vi "IEPE - Continuous  Input_tet.vi"() -> ()   [LabVIEW 2025]
doc: "This example demonstrates how to continuously acquire buffered acceleration, sound pressure, or force measurements from IEPE sensors using a DAQmx device.\n\nFor instructions on how to connect your signals to the DAQ device, refer to your device documentation."
uses:
  <vilib>/Math Plots/3D Math Plots/3D Contour/3D Contour XCtrl/3D Contour.xctl
  <vilib>/Utility/error.llb/DialogType.ctl
  <vilib>/DAQmx/read.llb/DAQmx Read (Analog 1D Wfm NChan NSamp).vi
  <extravilib>/ChannelInstances/Tag-bool/Read With Abort.vi
  <extravilib>/ChannelInstances/Tag-bool/Write With Abort.vi
  <vilib>/DAQmx/create/channels.llb/DAQmx Create Channel (AI-Acceleration-Accelerometer).vi
  <vilib>/DAQmx/miscellaneous.llb/DAQmx Fill In Error Info.vi
  <extravilib>/ChannelInstances/Tag-bool/Instantiate.vi
  <extravilib>/ChannelInstances/Tag-bool/EndpointRead.vi
  <vilib>/Waveform/WDTOps.llb/WDT Append Waveforms DBL.vi
  <extravilib>/ChannelInstances/Tag-bool/Endpoint.vi
  <vilib>/DAQmx/configure/timing.llb/DAQmx Timing (Sample Clock).vi
  <vilib>/DAQmx/configure/task.llb/DAQmx Configure Logging (TDMS).vi
  <vilib>/DAQmx/create/channels.llb/DAQmx Create Channel (AI-Sound Pressure-Microphone).vi
  <vilib>/DAQmx/create/channels.llb/DAQmx Create Channel (AI-Force-IEPE Sensor).vi
  <vilib>/DAQmx/configure/trigger.llb/DAQmx Start Trigger (Analog Edge).vi
  <vilib>/DAQmx/configure/trigger.llb/DAQmx Start Trigger (Time).vi
  <vilib>/DAQmx/configure/trigger.llb/DAQmx Start Trigger (Digital Edge).vi
  <vilib>/Waveform/WDTOps.llb/WDT Waveform Duration DBL.vi
  <resource>/objmgr/daqmx.rc
  <extravilib>/ChannelInstances/Tag-bool.lvlib
panel:
  out "_Vib3_3D-Kontur 3":refnum<class "3D Plot Datatype.lvclass">[](xcontrol)
  out "_Vib2_3D-Kontur":refnum<class "3D Plot Datatype.lvclass">[](xcontrol)
  in  "last order plot":sgl
  in  "rotation speed":sgl
  out "_Vib1_3D-Kontur":refnum<class "3D Plot Datatype.lvclass">[](xcontrol)
  in  "filename":string
  in  "Root folder":path
  in  "on hold time (s)":u32=900
  out "FFT":cluster{dbl, "freq_step":dbl, "abs_FFT":dbl[]}[](graph)
  in  "duration (s) control":dbl=30.0
  out "current duration":dbl caption="Dauer" format="%0.2f"
  in  "Trigger Type":T1(tab)
  in  "Digital Start Trigger Edge":i32(ring)=10280 caption="Edge" items=["Rising"=10280, "Falling"=10171]
  in  "Digital Start Trigger Source":tag="/Dev1/PFI0" caption="Source"
  in  "Digital Pause Trigger Pause When":i32(ring)=10192 caption="Pause When" items=["High"=10192, "Low"=10214]
  in  "Digital Pause Trigger Source":tag="/Dev1/PFI0" caption="Source"
  in  "Analog Start Trigger Level":dbl caption="Level" format="%0.2f"
  in  "Analog Start Trigger Hysteresis":dbl caption="Hysteresis" format="%.2f"
  in  "Analog Start Trigger Slope":i32(ring)=10280 caption="Slope" items=["Rising"=10280, "Falling"=10171]
  in  "Analog Start Trigger Source":string="APFI0" caption="Source"
  in  "Analog Pause Trigger Source":string="APFI0" caption="Source"
  in  "Analog Pause Trigger Pause When":i32(ring)=10093 caption="Pause When" items=["Above Level"=10093, "Below Level"=10107]
  in  "Analog Pause Trigger Level":dbl caption="Level" format="%.2f"
  in  "When":timestamp
  in  "Select Time\nManually":bool
  in  "IEPE Current Value (A)":dbl=0.004
  in  "IEPE Excitation Source":i32(ring)=10200 items=["Internal"=10200, "External"=10167, "None"=10230]
  in  "Terminal Configuration":i32(ring)=-1 items=["default"=-1, "RSE"=10083, "NRSE"=10078, "Differential"=10106, "Pseudodifferential"=12529]
  in  "Physical Channel":tag="cDAQ3Mod2/ai0"
  in  "Task Type":T2(tab)
  in  "Min Acceleration":dbl=-100.0
  in  "Max Acceleration":dbl=100.0
  in  "Sensitivity":dbl=50.0
  in  "Acceleration Units":i32(ring)=10186 items=["g"=10186, "m/s^2"=12470, "in/s^2"=12471, "From Custom Scale"=10065]
  in  "Sensitivity Units":i32(ring)=12509 items=["mVolts/g"=12509, "Volts/g"=12510]
  in  "Max Sound Pressure Level (dB)":dbl=120.0
  in  "Sound Pressure Units":i32(ring)=10081 items=["Pascals"=10081, "From Custom Scale"=10065]
  in  "Microphone Sensitivity":dbl=10.0
  in  "Sensitivity":dbl=50.0
  in  "Min Force":dbl=-100.0
  in  "Max Force":dbl=100.0
  in  "Sensitivity Units":i32(ring)=15891 items=["mVolts/N"=15891, "mVolts/lb"=15892]
  in  "Force Units":i32(ring)=15875 items=["Newtons"=15875, "Pounds"=15876, "From Custom Scale"=10065]
  in  "Stop":bool
  out "Waveform Graph":waveform(dbl)[](graph)
  in  "TDMS File Path":path
  in  "Samples per Loop":i32=100
  in  "Sample Rate":dbl=1000.0
  in  "Sample Clock Source":tag="OnboardClock"
  out "Actual Sample Rate":dbl=1000.0000111176631 format="%0.2f"
  in  "Logging Mode":i32(ring)=10231 items=["Off"=10231, "Log and Read"=15842]
  # "Channel Settings"
  # "Acquired Data"
  # "Trigger Settings"
  # "Timing Settings"
  # "Logging Settings"
  # "To enable triggers, select a tab above, and configure the settings.\n\nNot all hardware supports all trigger types. Refer to your device documentation for more information."
  # "This trigger type is not supported in continuous sample timing. \n\nRefer to your device documentation for more information on which triggers are supported."
  # "This trigger type is not supported in continuous sample timing. \n\nRefer to your device documentation for more information on which triggers are supported."
  # "If time is not manually set, task will begin after 10 seconds"
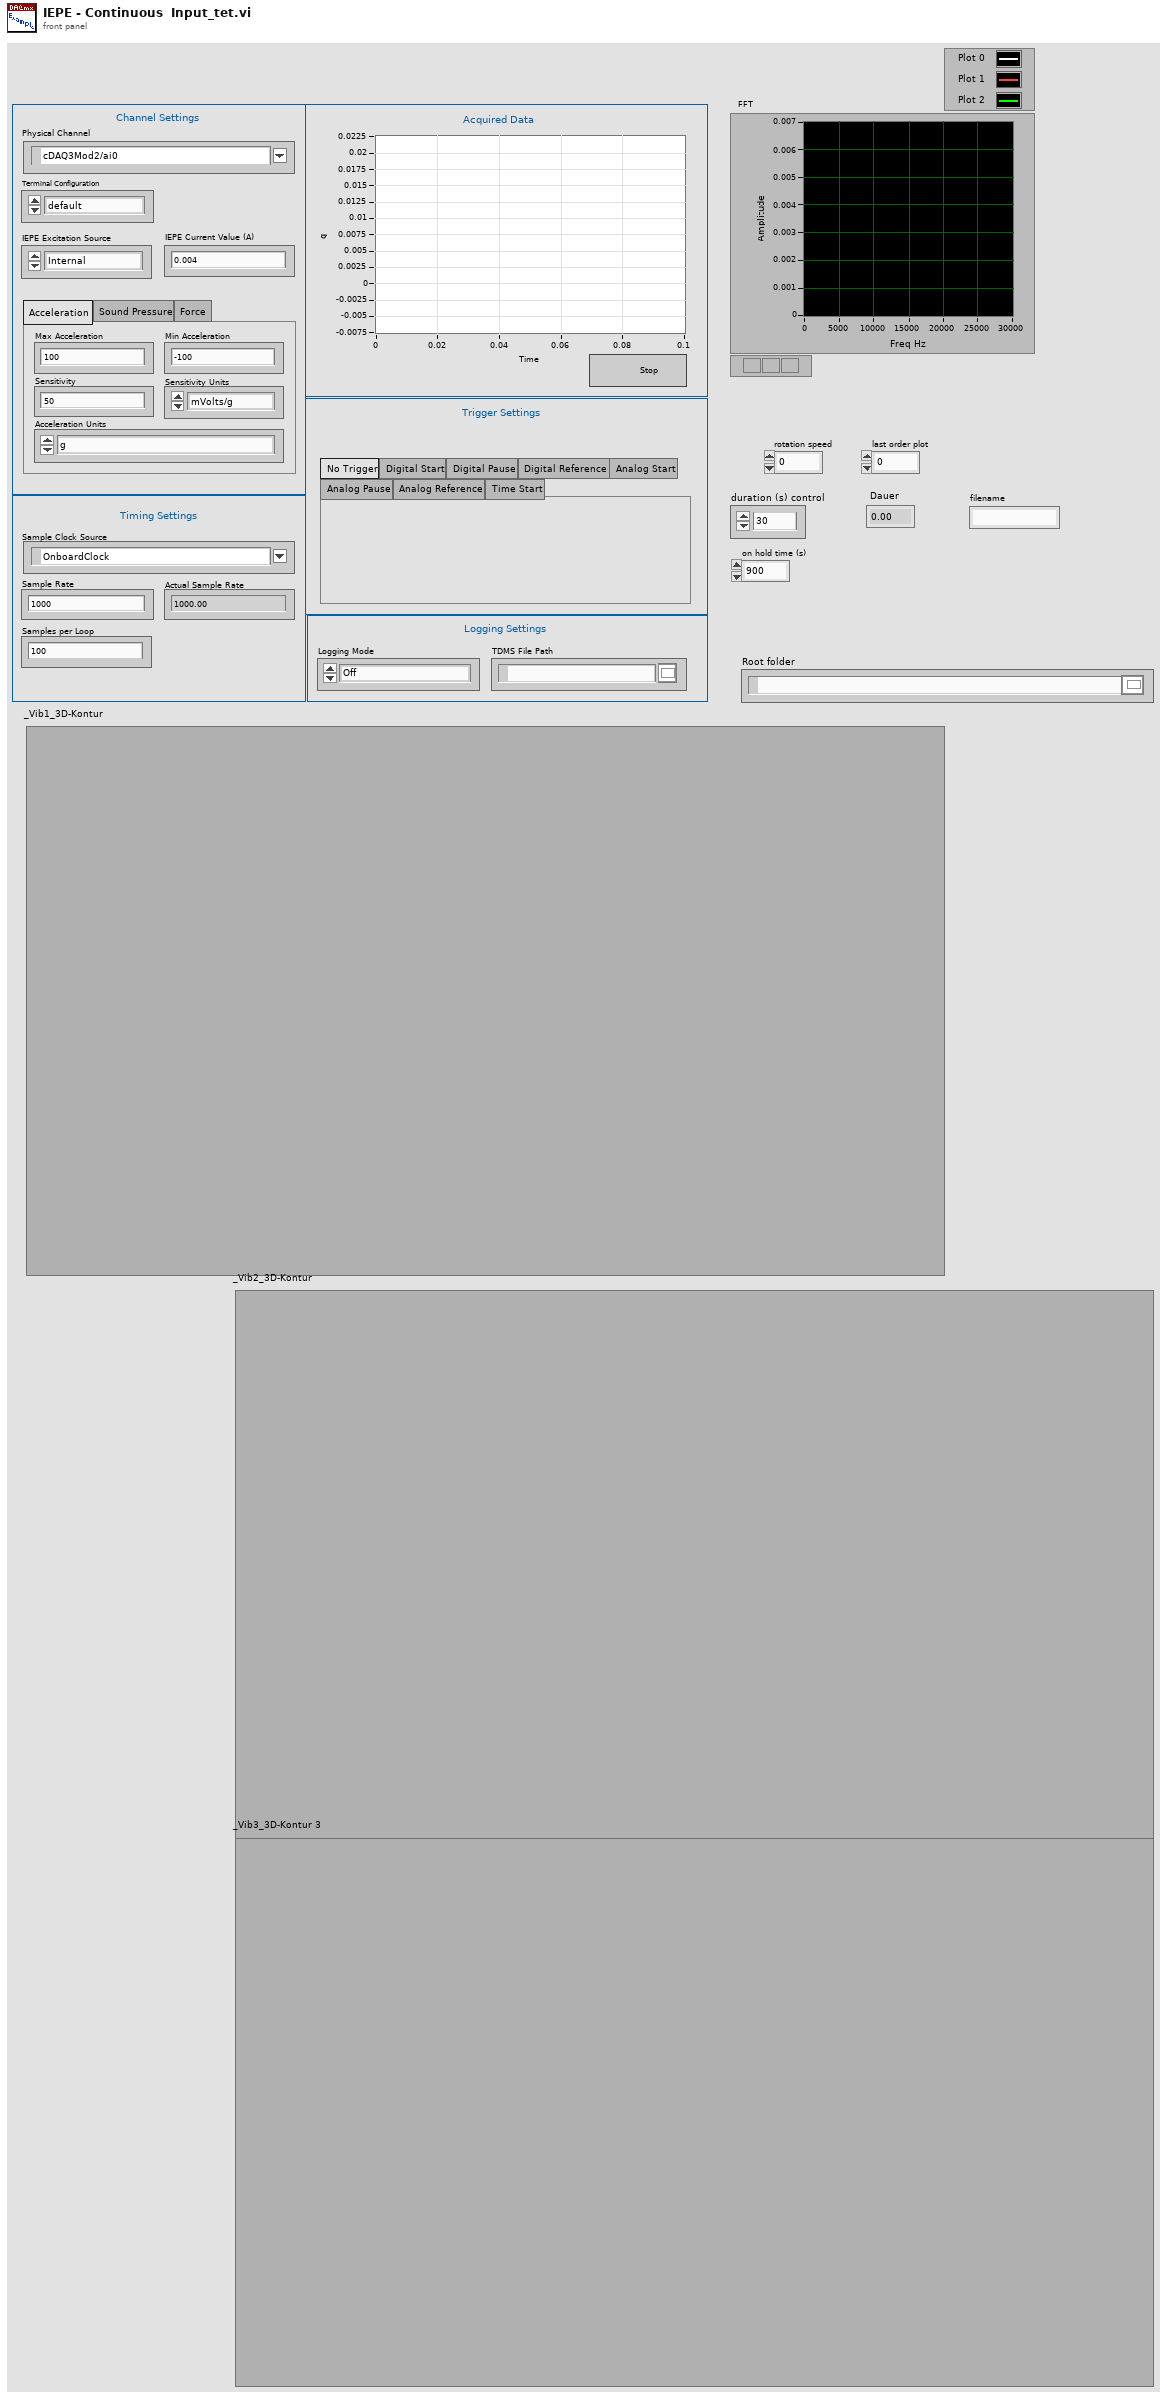
[diagram p1: front panel]
types:
  T1 = enum32{"No Trigger", "Digital Start", "Digital Pause", "Digital Reference", "Analog Start", "Analog Pause", "Analog Reference", "Time Start"}
  T2 = enum32{"Acceleration", "Sound Pressure", "Force"}
  T3 = cluster{"abs_FFT":dbl[], "frequencies":dbl[], "Huell_spec":dbl[], "Envelope":dbl[], "freq_step":dbl, "duration":dbl}
  T4 = typedef "DialogType.ctl" = u16
  T5 = cluster{"abs_FFT":dbl[], "frequencies":dbl[], "Huell_spec":dbl[], "Envelope":dbl[], "freq_step":dbl, "duration":dbl}[]
  T6 = typedef "Tag-bool.lvlib/))Channel.ctl" = refnum<queue>
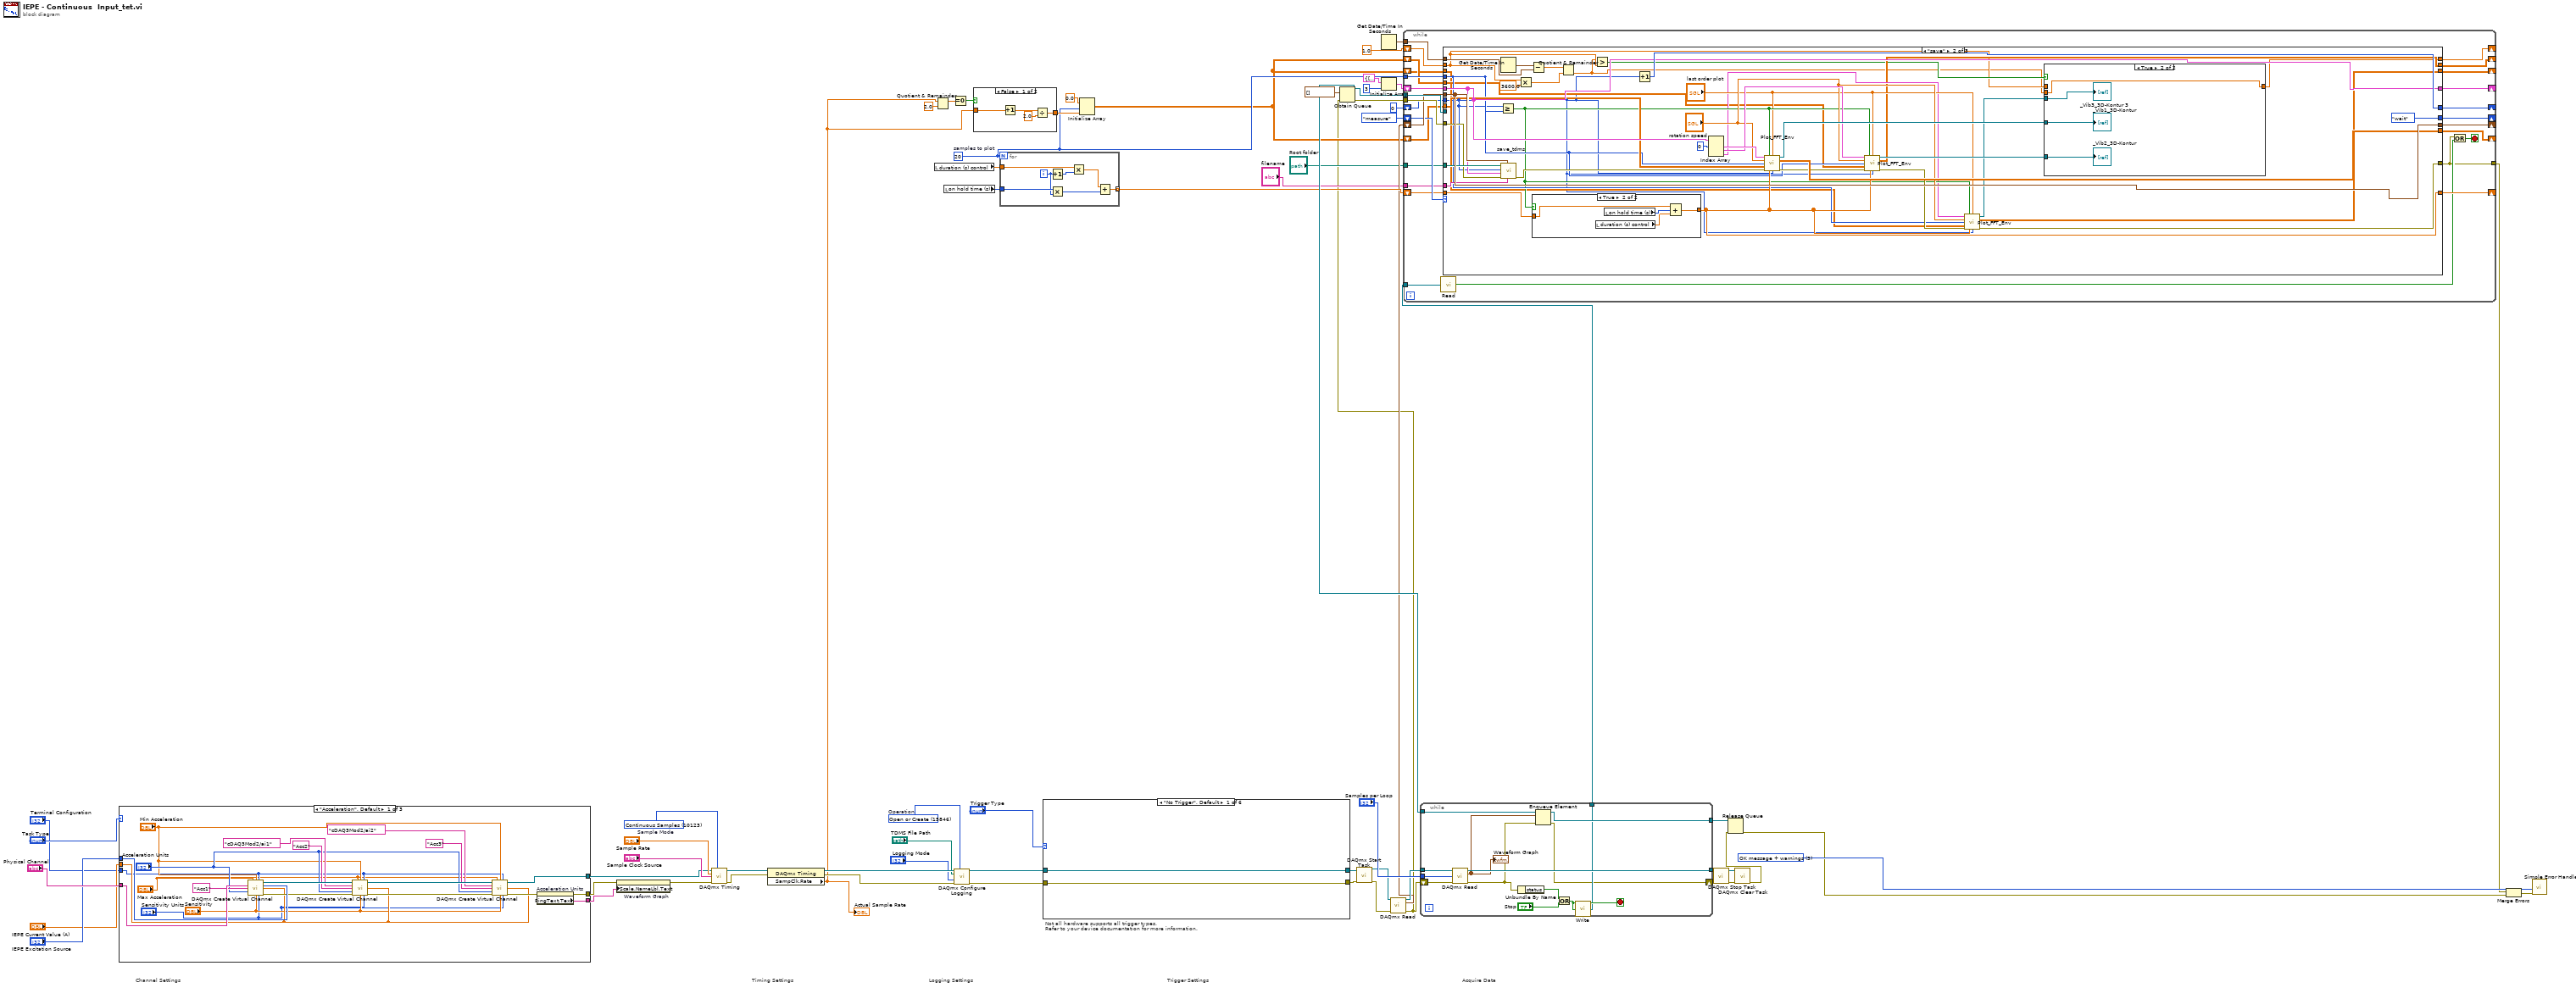
[diagram p0: block diagram]
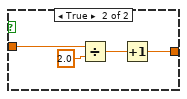
[diagram p2: hidden frame]
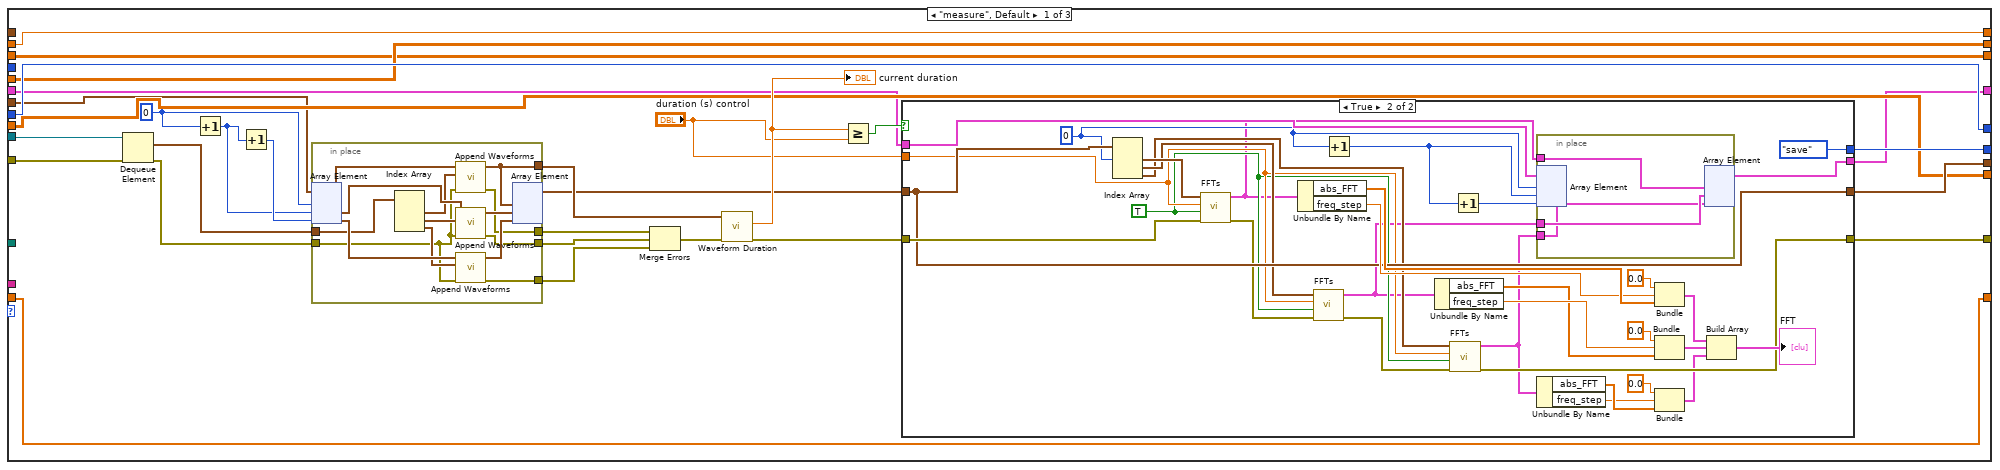
[diagram p3: hidden frame]
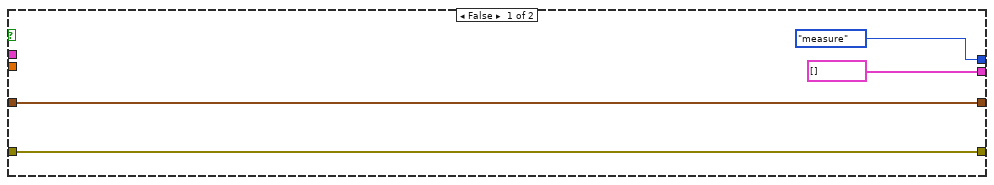
[diagram p4: hidden frame]
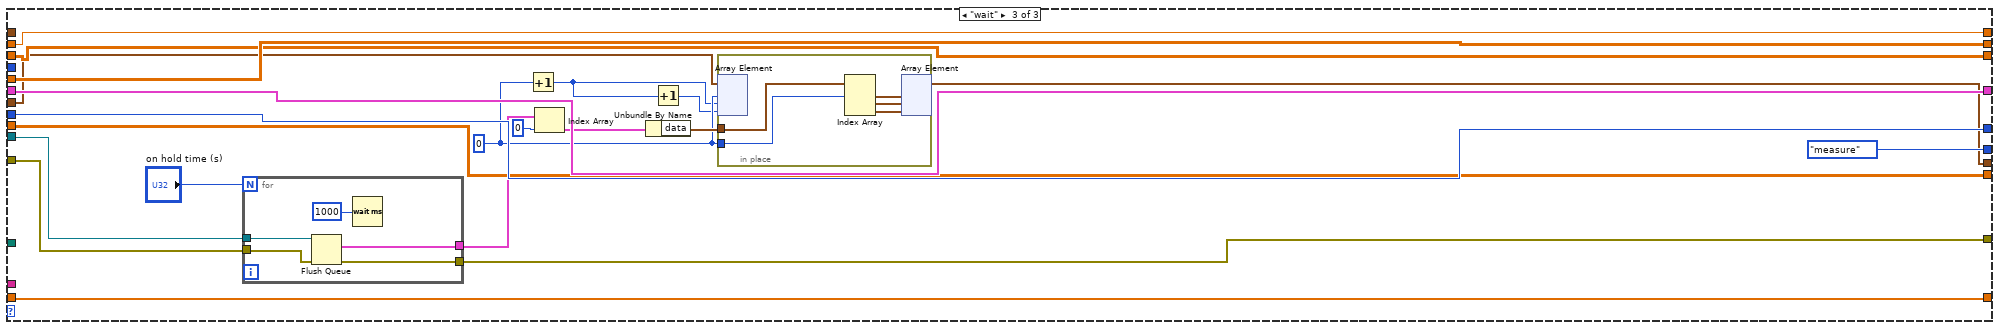
[diagram p7: hidden frame]
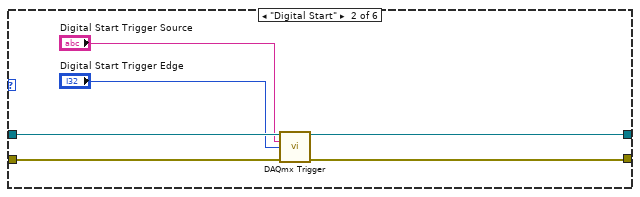
[diagram p8: hidden frame]
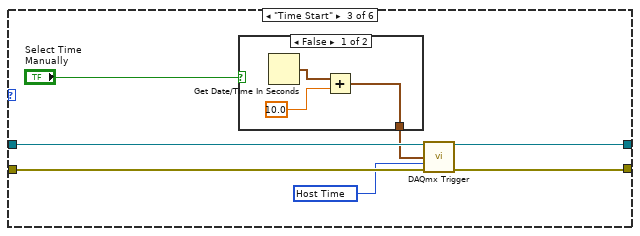
[diagram p9: hidden frame]
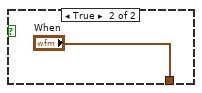
[diagram p10: hidden frame]
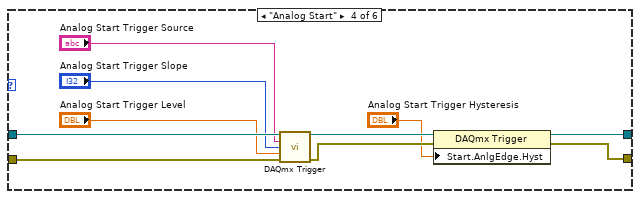
[diagram p11: hidden frame]
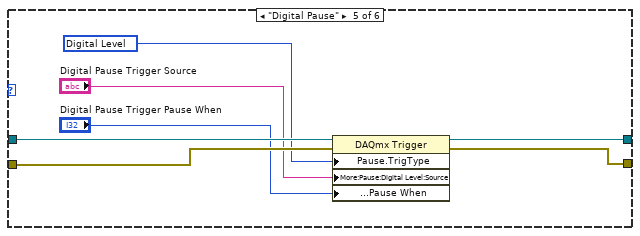
[diagram p12: hidden frame]
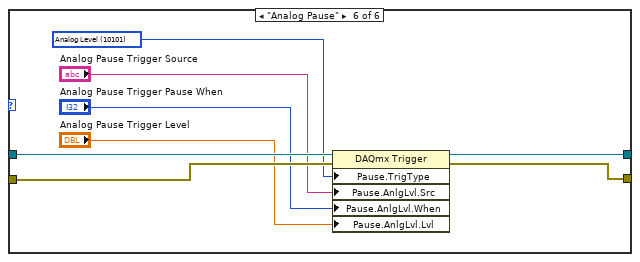
[diagram p13: hidden frame]
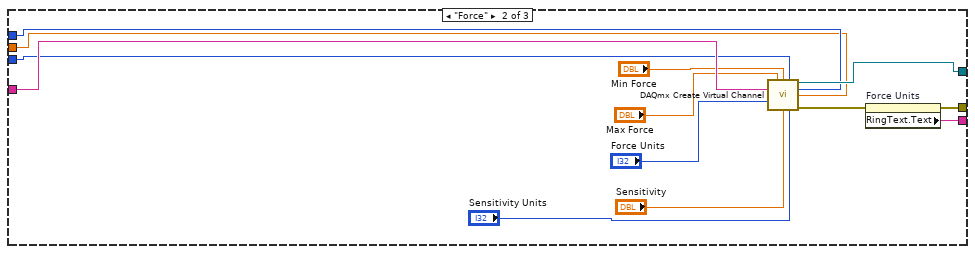
[diagram p14: hidden frame]
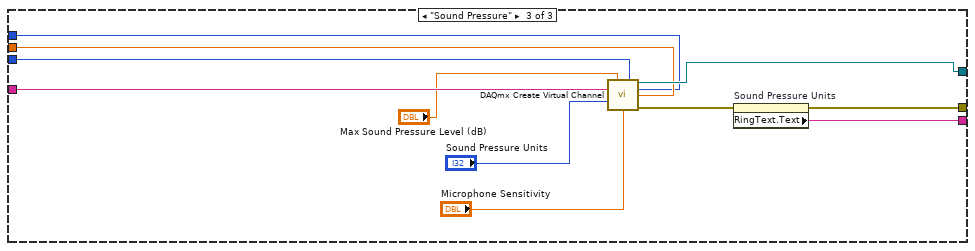
[diagram p15: hidden frame]
diagram:
  w14 = 20  # samples to plot
  w41 = T4 3 items=["no dialog", "OK message", "continue or stop message", "OK message + warnings", "continue/stop + warnings"] ("type of dialog (OK msg:1)")
  w59 = 15846 items=["Open"=10437, "Open or Create"=15846, "Create or Replace"=15847, "Create"=15848]  # Operation
  w62 = 10123 items=["Finite Samples"=10178, "Continuous Samples"=10123, "Hardware Timed Single Point"=12522]  # Sample Mode
  # "Trigger Settings"
  # "Not all hardware supports all trigger types.\nRefer to your device documentation for more information."
  # "Acquire Data"
  # "Timing Settings"
  # "Channel Settings"
  # "Logging Settings"
  n1 = case shown="\"Acceleration\", Default" "Task Type" {
    tunnel: [w84 w89 w103] -> w48
    tunnel: [w77 w99 w110] -> w49
    tunnel: "Physical Channel" -> [w86 w98 w109]
    tunnel: "IEPE Excitation Source" -> [w85 w97 w105]
    tunnel: "IEPE Current Value (A)" -> [w73 w96 w106]
    tunnel: "Terminal Configuration" -> [w66 w95 w108]
    tunnel: [w83 w88 w102] -> w47
    frame "Acceleration", Default {
      n2 = call-poly <vilib>:"DAQmx Create Virtual Channel.vi"("maximum value"="Max Acceleration", "minimum value"="Min Acceleration", "input terminal configuration"=w66, "physical channels"=w86, "current excitation source"=w85, "name to assign"="Acc1", "current excitation value"=w73, "units"="Acceleration Units", "sensitivity"="Sensitivity", "sensitivity units"="Sensitivity Units") -> ("task out"=w81:refnum<k21>, "error out"=w80:errorcluster)  [unwired: 4 in]
      n3 = call-poly <vilib>:"DAQmx Create Virtual Channel.vi"("task in"=w81, "maximum value"="Max Acceleration", "minimum value"="Min Acceleration", "input terminal configuration"=w66, "physical channels"=tag "cDAQ3Mod2/ai1" ("Physical Channel 2"), "name to assign"="Acc2", "current excitation value"=w73, "units"="Acceleration Units", "error in"=w80, "sensitivity"="Sensitivity", "sensitivity units"="Sensitivity Units") -> ("task out"=w79:refnum<k21>, "error out"=w78:errorcluster)  [unwired: 3 in]
      n4 = call-poly <vilib>:"DAQmx Create Virtual Channel.vi"("task in"=w79, "maximum value"="Max Acceleration", "minimum value"="Min Acceleration", "input terminal configuration"=w66, "physical channels"=tag "cDAQ3Mod2/ai2" ("Physical Channel 2"), "name to assign"="Acc3", "current excitation value"=w73, "units"="Acceleration Units", "error in"=w78, "sensitivity"="Sensitivity", "sensitivity units"="Sensitivity Units") -> ("task out"=w77:refnum<k21>, "error out"=w76:errorcluster)  [unwired: 3 in]
      n5 = property on="Acceleration Units" class="Ring (strict)"(error in=w76) -> (error out=w84:errorcluster, "RingText.Text"=w83:string)  [unwired: 1 in, 1 out]
    }
    frame "Force" {
      n6 = call-poly <vilib>:"DAQmx Create Virtual Channel.vi"("maximum value"="Max Force", "minimum value"="Min Force", "input terminal configuration"=w95, "physical channels"=w98, "current excitation source"=w97, "current excitation value"=w96, "units"="Force Units", "sensitivity"="Sensitivity", "sensitivity units"="Sensitivity Units") -> ("task out"=w99:refnum<k21>, "error out"=w87:errorcluster)  [unwired: 5 in]
      n7 = property on="Force Units" class="Ring (strict)"(error in=w87) -> (error out=w89:errorcluster, "RingText.Text"=w88:string)  [unwired: 1 in, 1 out]
    }
    frame "Sound Pressure" {
      n8 = call-poly <vilib>:"DAQmx Create Virtual Channel.vi"("maximum sound pressure level"="Max Sound Pressure Level (dB)", "input terminal configuration"=w108, "physical channels"=w109, "current excitation source"=w105, "current excitation value"=w106, "units"="Sound Pressure Units", "microphone sensitivity"="Microphone Sensitivity") -> ("task out"=w110:refnum<k21>, "error out"=w101:errorcluster)  [unwired: 7 in]
      n9 = property on="Sound Pressure Units" class="Ring (strict)"(error in=w101) -> (error out=w103:errorcluster, "RingText.Text"=w102:string)  [unwired: 1 in, 1 out]
    }
  }
  n10 = property on="Waveform Graph" class="WFGraph (strict)"(error in=w48, "YScale.NameLbl.Text"=w47) -> (error out=w46:errorcluster)  [unwired: 1 in, 1 out]
  n11 = call-poly <vilib>:"DAQmx Timing.vi"("task/channels in"=w49, "sample mode"=w62, "rate"="Sample Rate", "source"="Sample Clock Source", "error in"=w46) -> ("task out"=w64:refnum<k21>, "error out"=w63:errorcluster)  [unwired: 9 in]
  n12 = property class="DAQmx Timing"(reference=w64, error in=w63) -> (reference out=w61:refnum<k21>, error out=w60:errorcluster, "SampClk.Rate"=w24:dbl)
  "Actual Sample Rate" <- w24
  n13 = local read "duration (s) control"() -> (w16:dbl)
  n14 = Quotient & Remainder(x=w24, y=2.0) -> (x-y*floor(x/y)=w25:dbl)  [unwired: 1 out]
  n15 = local read "on hold time (s)"() -> (w17:u32)
  n16 = Equal To 0?(x=w25) -> (x = 0?=w26:bool)
  n17 = call-poly <vilib>:"DAQmx Configure Logging.vi"("task/channels in"=w61, "operation"=w59, "file path"="TDMS File Path", "logging mode"="Logging Mode", "error in"=w60) -> ("task out"=w38:refnum<k21>, "error out"=w39:errorcluster)  [unwired: 9 in]
  n18 = case shown="False" w26 {
    tunnel: w24 -> [w113 w116]
    tunnel: [w111 w115] -> w23
    frame False {
      n19 = Increment(x=w113) -> (x+1=w112:dbl)
      n20 = Divide(x=w112, y=2.0) -> (x/y=w111:dbl)
    }
    frame True {
      n21 = Divide(x=w116, y=2.0) -> (x/y=w118:dbl)
      n22 = Increment(x=w118) -> (x+1=w115:dbl)
    }
  }
  n23 = for {
    N: w14 -> [_]
    tunnel: w17 -> [w125]
    tunnel: w16 -> [w122]
    tunnel: [w119] -> w15 mode=indexing
    i -> [w124]
    n24 = Increment(x=w124) -> (x+1=w123:i32)
    n25 = Multiply(x=w125, y=w124) -> (x*y=w120:u32)
    n26 = Multiply(x=w122, y=w123) -> (x*y=w121:dbl)
    n27 = Add(x=w121, y=w120) -> (x+y=w119:dbl)
  }
  n28 = case shown="\"No Trigger\", Default" "Trigger Type" {
    tunnel: w38 -> [w127 w133 w140 w154 w161 w169]
    tunnel: w39 -> [w126 w132 w139 w153 w158 w166]
    tunnel: [w127 w131 w138 w151 w160 w168] -> w36
    tunnel: [w126 w130 w137 w150 w159 w167] -> w37
    frame "No Trigger", Default {
    }
    frame "Digital Start" {
      n29 = call-poly <vilib>:"DAQmx Trigger.vi"("task/channels in"=w133, "source"="Digital Start Trigger Source", "edge"="Digital Start Trigger Edge", "error in"=w132) -> ("task out"=w131:refnum<k21>, "error out"=w130:errorcluster)  [unwired: 10 in]
    }
    frame "Time Start" {
      w134 = 16126 items=["Host Time"=16126, "I/O Device Time"=16127] ("timescale")
      n30 = case shown="False" "Select Time\nManually" {
        tunnel: [w142 "When"] -> w135
        frame False {
          n31 = Get Date/Time In Seconds() -> (seconds since 1Jan1904=w143:timestamp)
          n32 = Add(x=w143, y=10.0) -> (x+y=w142:timestamp)
        }
        frame True {
        }
      }
      n33 = call-poly <vilib>:"DAQmx Trigger.vi"("task/channels in"=w140, "when"=w135, "timescale"=w134, "error in"=w139) -> ("task out"=w138:refnum<k21>, "error out"=w137:errorcluster)  [unwired: 10 in]
    }
    frame "Analog Start" {
      n34 = call-poly <vilib>:"DAQmx Trigger.vi"("task/channels in"=w154, "source"="Analog Start Trigger Source", "slope"="Analog Start Trigger Slope", "level"="Analog Start Trigger Level", "error in"=w153) -> ("task out"=w149:refnum<k21>, "error out"=w148:errorcluster)  [unwired: 9 in]
      n35 = property class="DAQmx Trigger"(reference=w149, error in=w148, "Start.AnlgEdge.Hyst"="Analog Start Trigger Hysteresis") -> (reference out=w151:refnum<k21>, error out=w150:errorcluster)
    }
    frame "Digital Pause" {
      w157 = 10152 items=["Analog Level"=10101, "Analog Window"=10103, "Digital Level"=10152, "Digital Pattern"=10398, "None"=10230] ("Pause.TrigType")
      n36 = property class="DAQmx Trigger"(reference=w161, error in=w158, "Pause.TrigType"=w157, "More:Pause:Digital Level:Source"="Digital Pause Trigger Source", "More:Pause:Digital Level:Pause When"="Digital Pause Trigger Pause When") -> (reference out=w160:refnum<k21>, error out=w159:errorcluster)
    }
    frame "Analog Pause" {
      w165 = 10101 items=["Analog Level"=10101, "Analog Window"=10103, "Digital Level"=10152, "Digital Pattern"=10398, "None"=10230] ("Pause.TrigType")
      n37 = property class="DAQmx Trigger"(reference=w169, error in=w166, "Pause.TrigType"=w165, "Pause.AnlgLvl.Src"="Analog Pause Trigger Source", "Pause.AnlgLvl.When"="Analog Pause Trigger Pause When", "Pause.AnlgLvl.Lvl"="Analog Pause Trigger Level") -> (reference out=w168:refnum<k21>, error out=w167:errorcluster)
    }
  }
  n38 = Initialize Array(0.0 ("Element"), w14, w23) -> (w5:dbl[][])
  n39 = call <vilib>:"DAQmx Start Task.vi"("task/channels in"=w36, "error in"=w37) -> ("task out"=w31:refnum<k21>, "error out"=w30:errorcluster)  [unwired: 12 in]
  n40 = Get Date/Time In Seconds() -> (seconds since 1Jan1904=w2:timestamp)
  n41 = Initialize Array(T3 {"abs_FFT"=[], "frequencies"=[], "Huell_spec"=[], "Envelope"=[], "freq_step"=0.0, "duration"=0.0} ("output cluster"), 3 ("dimension size")) -> (w11:T5)
  n42 = call-poly <vilib>:"DAQmx Read.vi"("task/channels in"=w31, "error in"=w30) -> ("task out"=w29:refnum<k21>, "data"=w12:waveform(dbl)[], "error out"=w4:errorcluster)  [unwired: 11 in]
  n43 = Obtain Queue(element data type=waveform(dbl)[] [] ("data"), error in (no error)=w4) -> (queue out=w35:refnum<queue>, error out=w3:errorcluster)  [unwired: 3 in, 1 out]
  n44 = while {
    tunnel: w29 -> [w182]
    tunnel: [w179] -> w43
    tunnel: w35 -> [w175]
    tunnel: [w174] -> w34
    tunnel: "Samples per Loop" -> [w173]
    tunnel: [w172] -> w6
    shift-right: [w170] -> w42
    shift-left: w4 -> [w181]
    stop <- w180 stop-if-true
    n45 = call-poly <vilib>:"DAQmx Read.vi"("task/channels in"=w182, "number of samples per channel"=w173, "error in"=w181) -> ("task out"=w179:refnum<k21>, "data"=w176:waveform(dbl)[], "error out"=w171:errorcluster)  [unwired: 10 in]
    "Waveform Graph" <- w176
    n46 = Unbundle By Name(w171) -> ("status"=w178:bool)
    n47 = Enqueue Element(queue=w175, element=w176, error in (no error)=w171) -> (queue out=w174:refnum<queue>, error out=w170:errorcluster)  [unwired: 1 in, 1 out]
    n48 = Or(x=w178, y="Stop") -> (x .or. y?=w180:bool)
    n49 = call <extravilib>:"Write.vi"("element"=w180) -> ("channel"=w172:T6)  [unwired: 1 out]
  }
  n50 = while {
    tunnel: w35 -> [w210]
    tunnel: w3 -> [w209]
    shift-right: [w208] -> _
    shift-left: w12 -> [w207]
    shift-right: [w194] -> _
    shift-left: w11 -> [w202]
    shift-right: [w205] -> _
    shift-left: enum16{"measure", "save", "wait"}."measure" -> [w206]
    shift-right: [w203] -> _
    shift-left: 0 -> [w204]
    tunnel: [w191] -> w21
    tunnel: "Root folder" -> [w201]
    tunnel: "filename" -> [w200]
    shift-right: [w198] -> _
    shift-left: w5 -> [w199]
    tunnel: w14 -> [w196]
    shift-right: [w195] -> _
    shift-left: w15 -> [w197]
    tunnel: w6 -> [w193]
    shift-right: [w187] -> _
    shift-left: w5 -> [w189]
    shift-right: [w186] -> _
    shift-left: w5 -> [w188]
    tunnel: w2 -> [w185]
    shift-right: [w184] -> _
    shift-left: 1.0 -> [w183]
    stop <- w190 stop-if-true
    n51 = call <extravilib>:"Read.vi"("channel"=w193) -> ("element"=w192:bool)  [unwired: 1 in, 1 out]
    n52 = case shown="\"save\"" w206 {
      tunnel: w210 -> [w239 _ w361]
      tunnel: w209 -> [w238 w327 w362]
      tunnel: [w235 w330 w345] -> w208
      tunnel: [w234 w314 w357] -> w191
      tunnel: w207 -> [w227 w330 w350]
      tunnel: [w214 w322 w358] -> w194
      tunnel: [w232 enum16{"measure", "save", "wait"}."wait" enum16{"measure", "save", "wait"}."measure"] -> w205
      tunnel: w204 -> [w231 w302 w363]
      tunnel: [w231 w331 w363] -> w203
      tunnel: w202 -> [w215 w322 w358]
      tunnel: w201 -> [_ w328 _]
      tunnel: w200 -> [_ w329 _]
      tunnel: w199 -> [w230 w320 w355]
      tunnel: [w230 w319 w355] -> w198
      tunnel: w197 -> [w228 w324 w354]
      tunnel: w196 -> [_ w311 _]
      tunnel: [w228 w312 w354] -> w195
      tunnel: w189 -> [w213 w306 w353]
      tunnel: w188 -> [w212 w305 w352]
      tunnel: [w213 w304 w353] -> w187
      tunnel: [w212 w303 w352] -> w186
      tunnel: w185 -> [_ w300 _]
      tunnel: [w211 w295 w343] -> w184
      tunnel: w183 -> [w211 w294 w343]
      frame "measure", Default {
        w217 = 0
        n53 = Dequeue Element(queue=w239, error in (no error)=w238) -> (element=w226:waveform(dbl)[], error out=w225:errorcluster)  [unwired: 1 in, 2 out]
        n54 = Increment(x=w217) -> (x+1=w216:i32)
        n55 = Increment(x=w216) -> (x+1=w218:i32)
        n56 = in-place {
          in-place-border: w226 -> [w250]
          in-place-border: w225 -> [w244]
          in-place-border: [w243] -> w224
          in-place-border: [w242] -> w223
          in-place-border: [w241] -> w222
          in-place-border: [w240] -> w221
          n57 = in-place-array #1(w227, w217, w216, w218) -> (w253:waveform(dbl), w252:waveform(dbl), w251:waveform(dbl))
          n58 = Index Array(array=w250) -> (element #1=w249:waveform(dbl), element #2=w248:waveform(dbl), element #3=w247:waveform(dbl))  [unwired: 3 in]
          n59 = call-poly <vilib>:"Append Waveforms.vi"("error in (no error)"=w244, "waveform B"=w249, "waveform A"=w253) -> ("error out"=w242:errorcluster, "waveform out"=w243:waveform(dbl))  [unwired: 7 in]
          n60 = call-poly <vilib>:"Append Waveforms.vi"("error in (no error)"=w244, "waveform B"=w248, "waveform A"=w252) -> ("error out"=w241:errorcluster, "waveform out"=w246:waveform(dbl))  [unwired: 7 in]
          n61 = call-poly <vilib>:"Append Waveforms.vi"("error in (no error)"=w244, "waveform B"=w247, "waveform A"=w251) -> ("error out"=w240:errorcluster, "waveform out"=w245:waveform(dbl))  [unwired: 7 in]
          n62 = in-place-array #1(w243, w246, w245) -> (w219:waveform(dbl)[])  [unwired: 3 out]
        }
        n63 = Merge Errors(w223, w222, w221) -> (w220:errorcluster)
        n64 = call-poly <vilib>:"Waveform Duration.vi"("error in (no error)"=w220, "waveform in"=w224) -> ("error out"=w229:errorcluster, "duration"=w237:dbl)  [unwired: 7 in, 1 out]
        "current duration" <- w237
        n65 = Greater Or Equal?(x=w237, y="duration (s) control") -> (x >= y?=w236:bool)
        n66 = case shown="True" w236 {
          tunnel: w229 -> [w256 w287]
          tunnel: w219 -> [w257 w284]
          tunnel: [w257 w284] -> w235
          tunnel: [w256 w268] -> w234
          tunnel: "duration (s) control" -> [_ w279]
          tunnel: [enum16{"measure", "save", "wait"}."measure" enum16{"measure", "save", "wait"}."save"] -> w232
          tunnel: w215 -> [_ w267]
          tunnel: [T5 [] w260] -> w214
          frame False {
          }
          frame True {
            w266 = 0 ("index")
            w278 = TRUE ("Envelope&Hu?")
            n67 = Index Array(array=w284, index #1=w266) -> (element #1=w283:waveform(dbl), element #2=w282:waveform(dbl), element #3=w271:waveform(dbl))  [unwired: 2 in]
            n68 = call "FFTs.vi"("error in"=w287, "Envelope&Hu?"=w278, "duration"=w279, "waveform in"=w283) -> ("error out"=w281:errorcluster, "output cluster"=w263:T3)  [unwired: 6 in]
            n69 = Unbundle By Name(w263) -> ("abs_FFT"=w289:dbl[], "freq_step"=w286:dbl)
            n70 = call "FFTs.vi"("error in"=w281, "Envelope&Hu?"=w278, "duration"=w279, "waveform in"=w282) -> ("error out"=w280:errorcluster, "output cluster"=w259:T3)  [unwired: 6 in]
            n71 = Increment(x=w266) -> (x+1=w265:i32)
            n72 = Unbundle By Name(w259) -> ("abs_FFT"=w276:dbl[], "freq_step"=w277:dbl)
            n73 = call "FFTs.vi"("error in"=w280, "Envelope&Hu?"=w278, "duration"=w279, "waveform in"=w271) -> ("error out"=w268:errorcluster, "output cluster"=w258:T3)  [unwired: 6 in]
            n74 = Increment(x=w265) -> (x+1=w264:i32)
            n75 = in-place {
              in-place-border: w263 -> [w292]
              in-place-border: w259 -> [w291]
              in-place-border: w258 -> [w290]
              n76 = in-place-array #2(w267, w266, w265, w264) -> ()  [unwired: 3 out]
              n77 = in-place-array #2(w292, w291, w290) -> (w260:T5)  [unwired: 3 out]
            }
            n78 = Unbundle By Name(w258) -> ("abs_FFT"=w275:dbl[], "freq_step"=w274:dbl)
            n79 = Bundle(0.0, "freq_step"=w286, "abs_FFT"=w289) -> (w270:cluster{dbl, "freq_step":dbl, "abs_FFT":dbl[]})  [unwired: 1 in]
            n80 = Bundle(0.0, "freq_step"=w277, "abs_FFT"=w276) -> (w262:cluster{dbl, "freq_step":dbl, "abs_FFT":dbl[]})  [unwired: 1 in]
            n81 = Bundle(0.0, "freq_step"=w274, "abs_FFT"=w275) -> (w261:cluster{dbl, "freq_step":dbl, "abs_FFT":dbl[]})  [unwired: 1 in]
            n82 = Build Array(w270, w262, w261) -> (→"FFT":cluster{dbl, "freq_step":dbl, "abs_FFT":dbl[]}[])
          }
        }
      }
      frame "save" {
        n83 = Greater Or Equal?(x=w302, y=w311) -> (x >= y?=w309:bool)
        n84 = Get Date/Time In Seconds() -> (seconds since 1Jan1904=w301:timestamp)
        n85 = call "save_tdms.vi"("filename"=w329, "waveform signal"=w330, "error in (no error)"=w327, "Array"=w322, "Numeric"=w302, "Folder with vibration"=w328) -> ("error out"=w326:errorcluster)  [unwired: 5 in]
        n86 = Multiply(x=w294, y=3600.0) -> (x*y=w296:dbl)
        n87 = Subtract(x=w301, y=w300) -> (x-y=w299:dbl)
        n88 = case shown="True" w309 {
          tunnel: w324 -> [w338 w342]
          tunnel: [w338 w341] -> w312
          frame False {
          }
          frame True {
            n89 = local read "duration (s) control"() -> (w339:dbl)
            n90 = local read "on hold time (s)"() -> (w340:u32)
            n91 = Compound Arithmetic op=ADD(w342, w340, w339) -> (w341:dbl[])
          }
        }
        n92 = Quotient & Remainder(x=w299, y=w296) -> (floor(x/y)=w293:dbl)  [unwired: 1 out]
        n93 = Greater?(x=w293, y=w294) -> (0:w298:bool)
        n94 = Increment(x=w302) -> (x+1=w331:i32)
        n95 = Index Array(array=w322, index #1=0 ("index")) -> (element #1=w321:T3, element #2=w318:T3, element #3=w307:T3)  [unwired: 2 in]
        n96 = call "Plot_FFT_Env.vi"("FFT input"=w321, "x > sample read?"=w309, "last order plot"="last order plot", "rotation speed"="rotation speed", "samples to plot"=w311, "Array in"=w320, "error in (no error)"=w326, "Array"=w312, "Numeric"=w302) -> ("3D Plot lvclass Array out"=w325:refnum<class "3D Plot Datatype.lvclass">[], "Array out"=w319:dbl[][], "error out"=w315:errorcluster)  [unwired: 4 in]
        n97 = call "Plot_FFT_Env.vi"("FFT input"=w318, "x > sample read?"=w309, "last order plot"="last order plot", "rotation speed"="rotation speed", "samples to plot"=w311, "Array in"=w306, "error in (no error)"=w315, "Array"=w312, "Numeric"=w302) -> ("3D Plot lvclass Array out"=w317:refnum<class "3D Plot Datatype.lvclass">[], "Array out"=w304:dbl[][], "error out"=w316:errorcluster)  [unwired: 4 in]
        n98 = call "Plot_FFT_Env.vi"("FFT input"=w307, "x > sample read?"=w309, "last order plot"="last order plot", "rotation speed"="rotation speed", "samples to plot"=w311, "Array in"=w305, "error in (no error)"=w316, "Array"=w312, "Numeric"=w302) -> ("3D Plot lvclass Array out"=w313:refnum<class "3D Plot Datatype.lvclass">[], "Array out"=w303:dbl[][], "error out"=w314:errorcluster)  [unwired: 4 in]
        n99 = case shown="True" w298 {
          tunnel: w325 -> [_ w337]
          tunnel: w317 -> [_ w336]
          tunnel: w313 -> [_ w335]
          tunnel: [w333 w334] -> w295
          tunnel: w294 -> [w333 _]
          tunnel: w293 -> [_ w334]
          frame False {
          }
          frame True {
            "_Vib1_3D-Kontur" <- w337
            "_Vib2_3D-Kontur" <- w336
            "_Vib3_3D-Kontur 3" <- w335
          }
        }
      }
      frame "wait" {
        w348 = 0 ("index")
        n100 = for {
          N: "on hold time (s)" -> [_]
          tunnel: w362 -> [w372]
          tunnel: w361 -> [w371]
          tunnel: [w370] -> w344
          tunnel: [w369] -> w357
          n101 = Flush Queue(queue=w371, error in (no error)=w372) -> (remaining elements=w370:cluster{"data":waveform(dbl)[]}[], error out=w369:errorcluster)  [unwired: 1 out]
          n102 = Wait (ms)(milliseconds to wait=u32 1000 ("Zu wartende ms")) -> ()  [unwired: 1 out]
        }
        n103 = Increment(x=w348) -> (x+1=w347:i32)
        n104 = Index Array(array=w344, index=0 ("Index")) -> (element=w351:cluster{"data":waveform(dbl)[]})
        n105 = Unbundle By Name(w351) -> ("data"=w349:waveform(dbl)[])
        n106 = Increment(x=w347) -> (x+1=w346:i32)
        n107 = in-place {
          in-place-border: w349 -> [w368]
          in-place-border: w348 -> [w367]
          n108 = in-place-array #3(w350, w348, w347, w346) -> ()  [unwired: 3 out]
          n109 = Index Array(array=w368, index #1=w367) -> (element #1=w366:waveform(dbl), element #2=w365:waveform(dbl), element #3=w364:waveform(dbl))  [unwired: 2 in]
          n110 = in-place-array #3(w366, w365, w364) -> (w345:waveform(dbl)[])  [unwired: 3 out]
        }
      }
    }
    n111 = Or(x=w191, y=w192) -> (x .or. y?=w190:bool)
  }
  n112 = call <vilib>:"DAQmx Stop Task.vi"("task/channels in"=w43, "error in"=w42) -> ("task out"=w45:refnum<k21>, "error out"=w44:errorcluster)  [unwired: 12 in]
  n113 = call <vilib>:"DAQmx Clear Task.vi"("task in"=w45, "error in"=w44) -> ("error out"=w33:errorcluster)  [unwired: 13 in]
  n114 = Release Queue(queue=w34, error in (no error)=w33) -> (error out=w20:errorcluster)  [unwired: 1 in, 2 out]
  n115 = Merge Errors(w21, w20) -> (w19:errorcluster)
  n116 = call <vilib>:"Simple Error Handler.vi"("type of dialog (OK msg:1)"=w41, "error in (no error)"=w19) -> ()  [unwired: 3 in, 5 out]
